vi "SRV_Sensor PARSE_#ND.vi"(0 "Return Data":string) -> (3 "Constant Command":string, 10 "Value":u8)   [LabVIEW 2009]
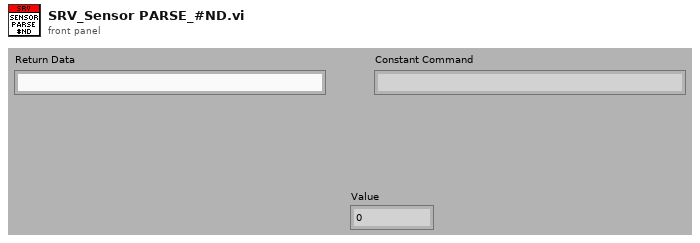
[diagram p1: front panel]
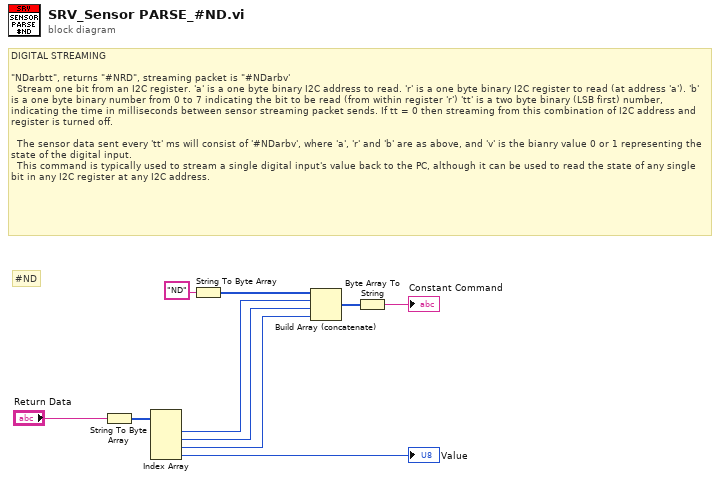
[diagram p0: block diagram]
diagram:
  # "#ND"
  # "DIGITAL STREAMING\n\n\"NDarbtt\", returns \"#NRD\", streaming packet is \"#NDarbv'\n  Stream one bit from an I2C register. 'a' is a one byte binary I2C address to read. 'r' is a one byte binary I2C register to read (at address 'a'). 'b' is a one byte binary number from 0 to 7 indicating the bit to be read (from within register 'r') 'tt' is a two byte binary (LSB first) number, indicating the time in milliseconds between sensor streaming packet sends. If tt = 0 then streaming from this combination of I2C address and register is turned off.\n\n  The sensor data sent every 'tt' ms will consist of '#NDarbv', where 'a', 'r' and 'b' are as above, and 'v' is the bianry value 0 or 1 representing the state of the digital input.\n  This command is typically used to stream a single digital input's value back to the PC, although it can be used to read the state of any single bit in any I2C register at any I2C address."
  n1 = String To Byte Array(string="Return Data") -> (unsigned byte array=w8:u8[])
  n2 = Index Array(array=w8) -> (element #1=w4:u8, element #2=w3:u8, element #3=w2:u8, element #4=→"Value":u8)  [unwired: 4 in]
  n3 = String To Byte Array(string="ND" ("format string")) -> (unsigned byte array=w5:u8[])
  n4 = Build Array (concatenate)(w5, w4, w3, w2) -> (w7:u8[])
  n5 = Byte Array To String(unsigned byte array=w7) -> (string=→"Constant Command":string)
